vi "Init.vi"(7 "Enclave":refnum<class "Enclave.lvclass">, 8 "error in (no error)":errorcluster, 11 "Tag DVR":refnum<data-value>) -> (0 "error out":errorcluster, 3 "Tag out":refnum<class "Tag.lvclass">)   [LabVIEW 2022 SP3, in "Enclave.lvlib" / "Tag.lvclass"]
uses:
  Tag.lvclass
  Enclave/Enclave.lvclass
  Tag Data.ctl
  Element.ctl
  Tag.lvclass/Tag.ctl
  Enclave.lvlib
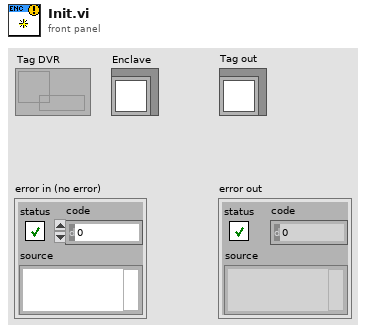
[diagram p1: front panel]
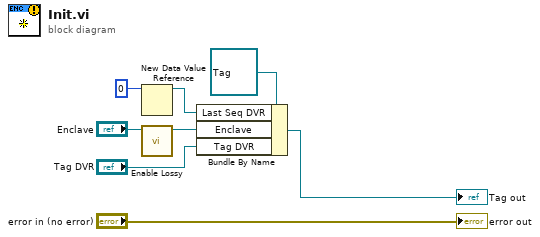
[diagram p0: block diagram]
diagram:
  n1 = New Data Value Reference(data value=u64 0) -> (data value reference=w2:refnum<data-value>)  [unwired: 1 in, 1 out]
  n2 = call "Enable Lossy.vi"("Enclave in"="Enclave") -> ("Enclave out"=w4:refnum<class "Enclave.lvclass">)  [unwired: 9 in, 1 out]
  n3 = Bundle By Name(cluster=refnum<class "Tag.lvclass"> refnum ("Tag in"), "Last Seq DVR"=w2, "Enclave"=w4, "Tag DVR"="Tag DVR") -> (→"Tag out":refnum<class "Tag.lvclass">)
  "error out" <- "error in (no error)"
